vi "Destroy.vi"(8 "error in (no error)":errorcluster, 11 "Configuration Manager In":refnum<class "Configuration Manager.lvclass">) -> (0 "error out":errorcluster)   [LabVIEW 2020, in "Configuration Manager.lvclass"]
uses:
  Configuration Manager.lvclass
  Configuration Manager.lvclass/Configuration Manager.ctl
  <vilib>/Utility/config.llb/NI_LVConfig.lvlib
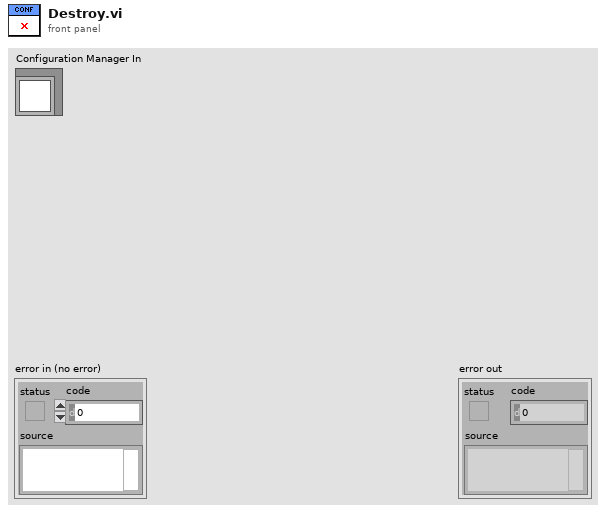
[diagram p1: front panel]
types:
  T1 = typedef "NI_LVConfig.lvlib/Config Data RefNum.ctl" = refnum<k1>
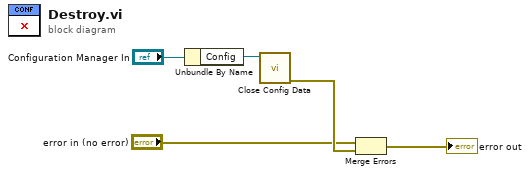
[diagram p0: block diagram]
diagram:
  n1 = Unbundle By Name("Configuration Manager In") -> ("Config"=w3:T1)
  n2 = call <vilib>:"Close Config Data.vi"("refnum"=w3) -> ("error out"=w4:errorcluster)  [unwired: 9 in, 1 out]
  n3 = Merge Errors("error in (no error)", w4) -> (→"error out":errorcluster)
